vi "Folders_Required.vi"(1 "No dialogs":bool, 2 "Filenames":path[](array[path]), 3 "Add _pp?":bool, 4 "New Root":path) -> (0 "Array":path[](array[path]))   [LabVIEW 2012]
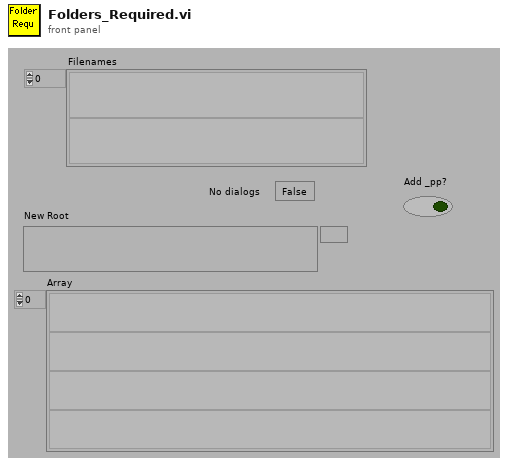
[diagram p1: front panel]
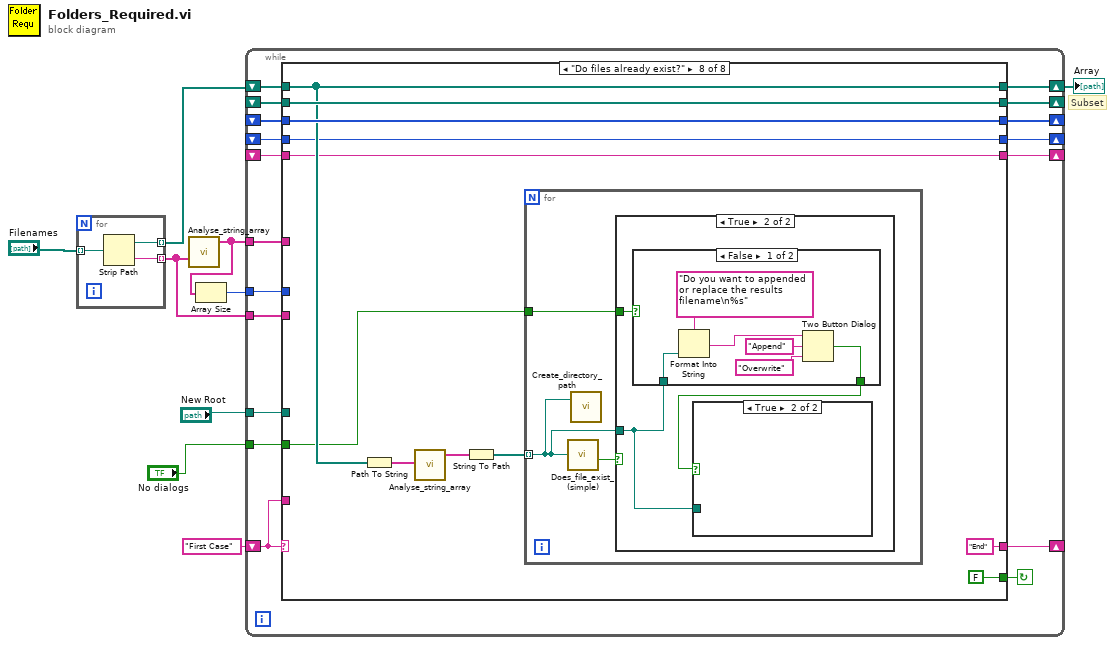
[diagram p0: block diagram]
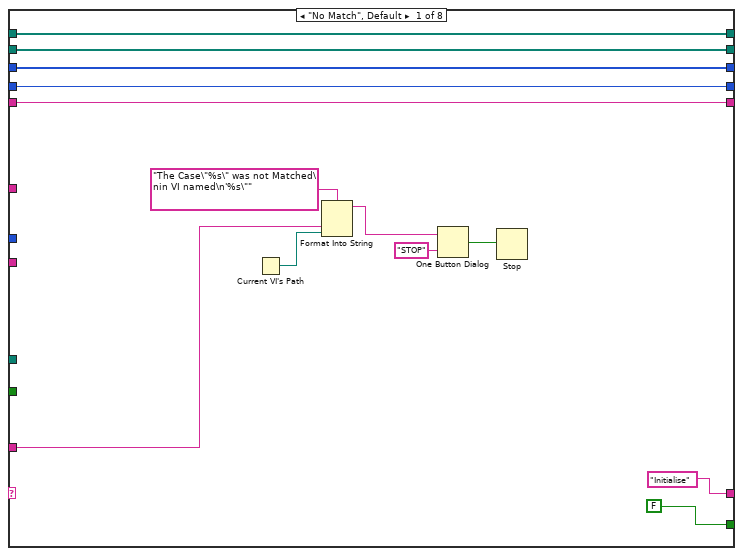
[diagram p2: hidden frame]
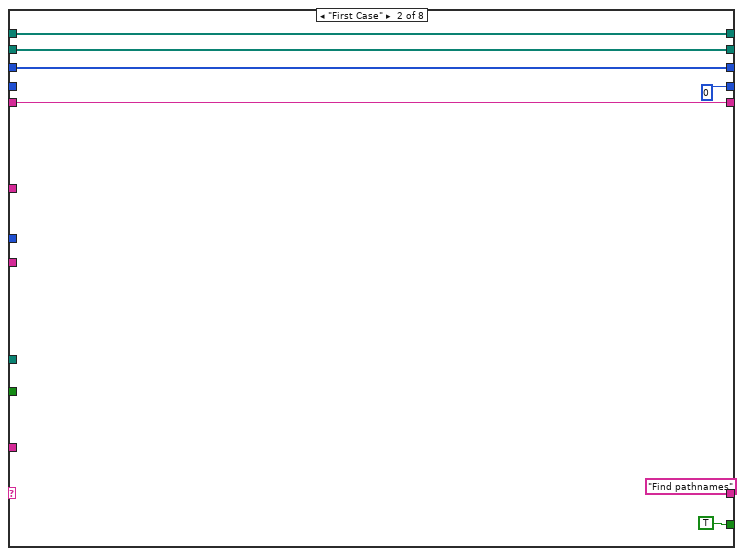
[diagram p3: hidden frame]
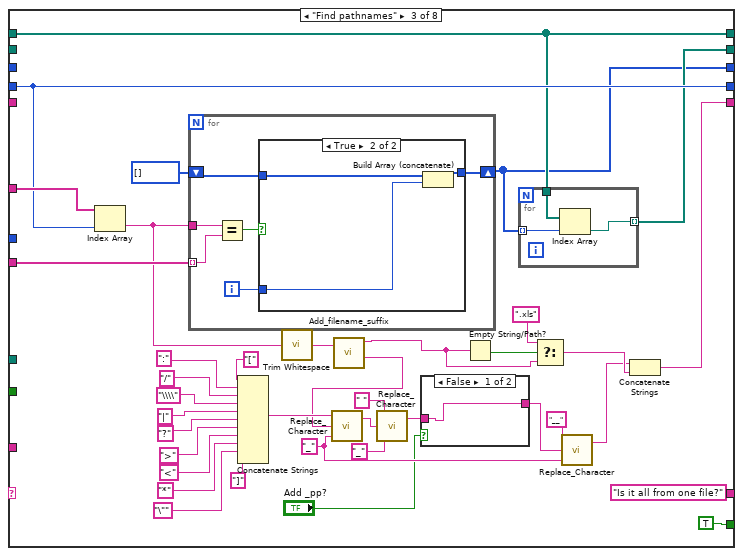
[diagram p4: hidden frame]
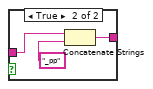
[diagram p5: hidden frame]
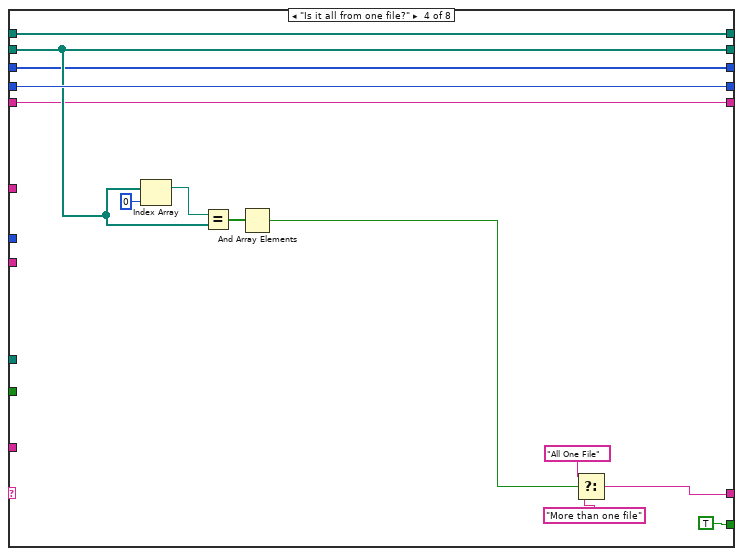
[diagram p7: hidden frame]
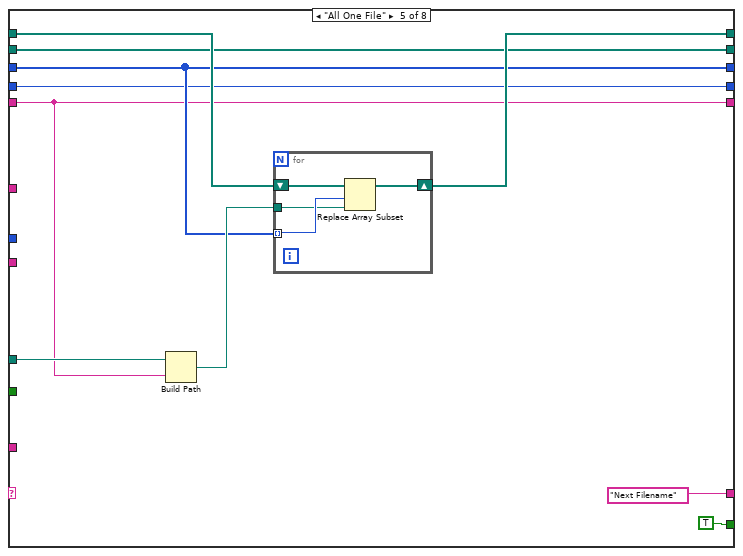
[diagram p8: hidden frame]
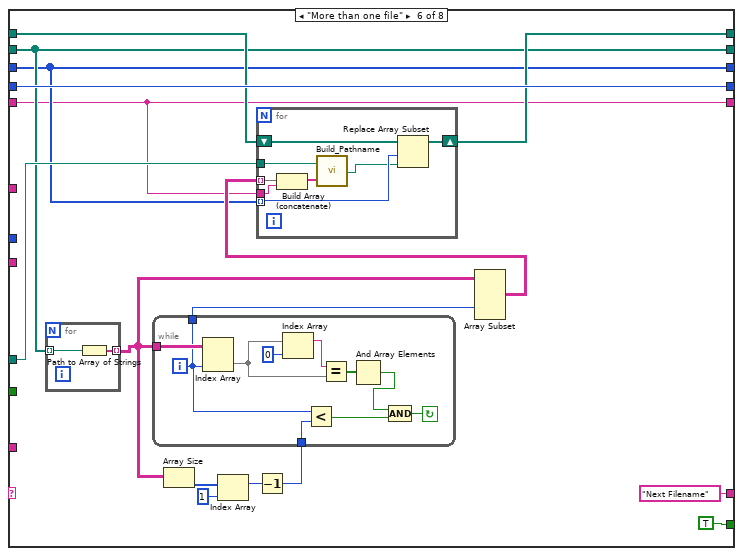
[diagram p9: hidden frame]
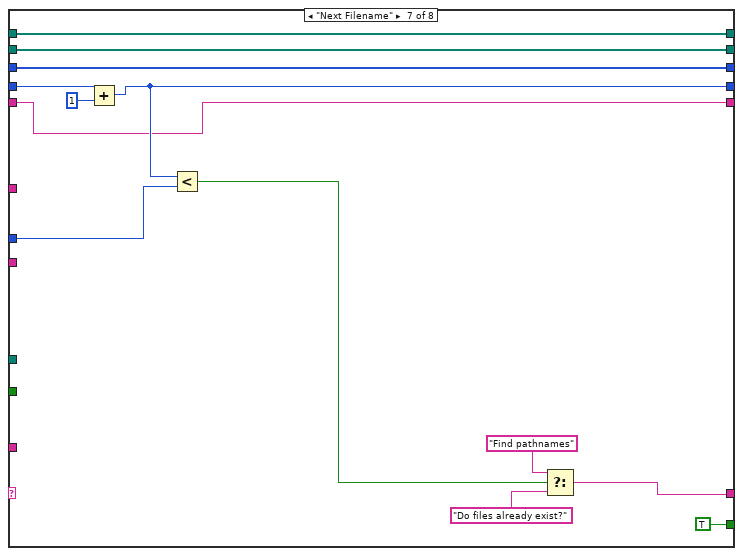
[diagram p10: hidden frame]
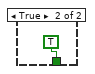
[diagram p12: hidden frame]
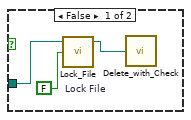
[diagram p13: hidden frame]
diagram:
  # "Subset"
  n1 = for {
    tunnel: "Filenames" -> [w12] mode=indexing
    tunnel: [w11] -> w8 mode=indexing
    tunnel: [w10] -> w2 mode=indexing
    n2 = Strip Path(path=w12) -> (stripped path=w10:path, name=w11:string)
  }
  n3 = call "Analyse_string_array.vi"("String array"=w8) -> ("Unique strings"=w6:string[])  [unwired: 2 out]
  n4 = Array Size(array=w6) -> (size(s)=w5:i32)
  n5 = while {
    shift-left: _ -> [w15]
    shift-right: [w14] -> _
    tunnel: w5 -> [w17]
    shift-left: w2 -> [w19]
    shift-right: [w20] -> w4
    tunnel: "New Root" -> [w21]
    tunnel: w8 -> [w22]
    tunnel: w6 -> [w23]
    shift-left: _ -> [w24]
    shift-right: [w26] -> _
    shift-left: _ -> [w25]
    shift-right: [w16] -> _
    shift-left: _ -> [w18]
    shift-right: [w27] -> _
    shift-left: "First Case" -> [w28]
    shift-right: [w29] -> _
    tunnel: "No dialogs" -> [w13]
    stop <- w30 continue-if-true
    n6 = case shown="\"Do files already exist?\"" w28 {
      tunnel: [FALSE TRUE TRUE TRUE TRUE TRUE TRUE FALSE] -> w30
      tunnel: ["Initialise" "Find pathnames" "Is it all from one file?" w113 "Next Filename" "Next Filename" w172 "End"] -> w29
      tunnel: w28 -> [w38 _ _ _ _ _ _ _]
      tunnel: [w34 w46 w81 w108 w123 w136 w181 w192] -> w27
      tunnel: [w33 0 w84 w117 w120 w147 w177 w186] -> w26
      tunnel: w25 -> [w32 w45 _ w107 w122 w135 w175 w191]
      tunnel: w24 -> [w33 _ w84 w117 w120 w147 w179 w186]
      tunnel: w23 -> [_ _ w86 _ _ _ _ _]
      tunnel: w22 -> [_ _ w85 _ _ _ _ _]
      tunnel: w21 -> [_ _ _ _ w127 w140 _ _]
      tunnel: [w35 w47 w82 w109 w124 w141 w180 w189] -> w20
      tunnel: w19 -> [w35 w47 w82 w109 w125 w142 w180 w189]
      tunnel: w18 -> [w34 w46 _ w108 w123 w136 w181 w192]
      tunnel: w17 -> [_ _ _ _ _ _ w176 _]
      tunnel: [w32 w45 w80 w107 w122 w135 w175 w191] -> w16
      tunnel: w15 -> [w31 w44 _ w106 w119 w133 w169 w184]
      tunnel: [w31 w44 w64 w106 w119 w133 w169 w184] -> w14
      tunnel: w13 -> [_ _ _ _ _ _ _ w182]
      frame "No Match", Default {
        n7 = Current VI's Path() -> (path=w37:path)
        n8 = Format Into String(format string="The Case\"%s\" was not Matched\nin VI named\n'%s\"" ("Format String"), w38, w37) -> (resulting string=w41:string)  [unwired: 2 in, 1 out]
        n9 = One Button Dialog(message=w41, button name ("OK")="STOP") -> (true=w39:bool)
        n10 = Stop(stop? (T)=w39) -> ()
      }
      frame "First Case" {
      }
      frame "Find pathnames" {
        w63 = "_" ("Replace with")
        n11 = Index Array(array=w86, index=w84) -> (element=w67:string)
        n12 = for {
          tunnel: w67 -> [w101]
          tunnel: w85 -> [w100] mode=indexing
          shift-right: [w97] -> w80
          shift-left: i32[] [] -> [w98]
          i -> [w96]
          n13 = Equal?(x=w101, y=w100) -> (x = y?=w99:bool)
          n14 = case shown="True" w99 {
            tunnel: w98 -> [w102 w105]
            tunnel: [w102 w104] -> w97
            tunnel: w96 -> [_ w103]
            frame False {
            }
            frame True {
              n15 = Build Array (concatenate)(w105, w103) -> (w104:i32[])
            }
          }
        }
        n16 = Concatenate Strings("[" ("Substring"), ":", "/", "\\\\", "|", "?", ">", "<", "*", "\"", "]" ("Substring")) -> (w68:string)
        n17 = call <vilib>:"Trim Whitespace.vi"("string"=w67) -> ("trimmed string"=w66:string)  [unwired: 1 in]
        n18 = call "Add_filename_suffix.vi"("Filename"=w66) -> ("Original Suffix"=w55:string, "Base name"=w65:string)  [unwired: 1 in, 2 out]
        n19 = call "Replace_Character.vi"("Replace with"=w63, "Input String"=w65, "Search For"=w68) -> ("Output string"=w59:string)  [unwired: 1 out]
        n20 = call "Replace_Character.vi"("Replace with"="_", "Input String"=w59, "Search For"=" ") -> ("Output string"=w60:string)  [unwired: 1 out]
        n21 = case shown="False" "Add _pp?" {
          tunnel: [w89 w91] -> w62
          tunnel: w60 -> [w89 w90]
          frame False {
          }
          frame True {
            n22 = Concatenate Strings(w90, "_pp" ("Substring")) -> (w91:string)
          }
        }
        n23 = Empty String/Path?(string/path=w55) -> (empty?=w56:bool)
        n24 = for {
          tunnel: w80 -> [w95] mode=indexing
          tunnel: w82 -> [w94]
          tunnel: [w93] -> w81 mode=indexing
          n25 = Index Array(array=w94, index=w95) -> (element=w93:path)
        }
        n26 = Select(t=".xls", s=w56, f=w55) -> (s? t:f=w54:string)
        n27 = call "Replace_Character.vi"("Replace with"=w63, "Input String"=w62, "Search For"="__") -> ("Output string"=w52:string)  [unwired: 1 out]
        n28 = Concatenate Strings(w52, w54) -> (w64:string)
      }
      frame "Is it all from one file?" {
        n29 = Index Array(array=w108, index=0 ("Index")) -> (element=w111:path)
        n30 = Equal?(x=w111, y=w108) -> (x = y?=w110:bool[])
        n31 = And Array Elements(Boolean array=w110) -> (logical AND=w116:bool)
        n32 = Select(t="All One File", s=w116, f="More than one file") -> (s? t:f=w113:string)
      }
      frame "All One File" {
        n33 = Build Path(base path=w127, name or relative path=w119) -> (appended path=w126:path)
        n34 = for {
          tunnel: w122 -> [w130] mode=indexing
          shift-right: [w131] -> w124
          shift-left: w125 -> [w132]
          tunnel: w126 -> [w129]
          n35 = Replace Array Subset(array=w132, new element=w129, index=w130) -> (w131:path[])
        }
      }
      frame "More than one file" {
        n36 = for {
          tunnel: w136 -> [w168] mode=indexing
          tunnel: [w167] -> w138 mode=indexing
          n37 = Path to Array of Strings(0:w168) -> (2:w167:string[])  [unwired: 1 out]
        }
        n38 = Array Size(array=w138) -> (size(s)=w145:i32[])
        n39 = Index Array(array=w145, index=1 ("Index")) -> (element=w144:i32)
        n40 = Decrement(x=w144) -> (x-1=w143:i32)
        n41 = while {
          tunnel: [w149] -> w139
          tunnel: w143 -> [w153]
          tunnel: w138 -> [w158]
          i -> [w149]
          stop <- w150 continue-if-true
          n42 = Index Array(array=w158, index (col)=w149) -> (element=w154:string[])  [unwired: 1 in]
          n43 = Index Array(array=w154, index=0 ("Index")) -> (element=w156:string)
          n44 = Less?(x=w149, y=w153) -> (x < y?=w152:bool)
          n45 = Equal?(x=w156, y=w154) -> (x = y?=w155:bool[])
          n46 = And Array Elements(Boolean array=w155) -> (logical AND=w151:bool)
          n47 = Compound Arithmetic op=AND(w151, w152) -> (w150:bool)
        }
        n48 = Array Subset(array=w138, index (col)=w139) -> (w137:string[][])  [unwired: 3 in]
        n49 = for {
          tunnel: w135 -> [w164] mode=indexing
          shift-right: [w165] -> w141
          shift-left: w142 -> [w166]
          tunnel: w140 -> [w163]
          tunnel: w137 -> [w161] mode=indexing
          tunnel: w133 -> [w159]
          n50 = Build Array (concatenate)(w161, w159) -> (w160:string[])
          n51 = call "Build_Pathname.vi"("PathElements"=w160, "PathnameIn"=w163) -> ("AppendedPath"=w162:path)
          n52 = Replace Array Subset(array=w166, new element=w162, index=w164) -> (w165:path[])
        }
      }
      frame "Next Filename" {
        n53 = Add(x=w179, y=1) -> (x+y=w177:i32)
        n54 = Less?(x=w177, y=w176) -> (x < y?=w174:bool)
        n55 = Select(t="Find pathnames", s=w174, f="Do files already exist?") -> (s? t:f=w172:string)
      }
      frame "Do files already exist?" {
        n56 = Path To String(path=w189) -> (string=w188:string[])
        n57 = call "Analyse_string_array.vi"("String array"=w188) -> ("Unique strings"=w183:string[])  [unwired: 2 out]
        n58 = String To Path(string=w183) -> (path=w187:path[])
        n59 = for {
          tunnel: w187 -> [w194] mode=indexing
          tunnel: w182 -> [w193]
          n60 = call "Does_file_exist_(simple).vi"("Pathname"=w194) -> ("exists?"=w195:bool)
          n61 = call "Create_directory_path.vi"("Path name"=w194) -> ()  [unwired: 1 in, 2 out]
          n62 = case shown="True" w195 {
            tunnel: w194 -> [_ w197]
            tunnel: w193 -> [_ w196]
            frame False {
            }
            frame True {
              n63 = case shown="False" w196 {
                tunnel: [w200 TRUE ("T button?")] -> w198
                tunnel: w197 -> [w199 _]
                frame False {
                  n64 = Format Into String(format string="Do you want to appended or replace the results filename\n%s" ("Format String"), w199) -> (resulting string=w203:string)  [unwired: 2 in, 1 out]
                  n65 = Two Button Dialog(message=w203, 1:"Overwrite" ("F button name (\"Cancel\")"), 2:"Append" ("T button name (\"OK\")")) -> (T button?=w200:bool)
                }
                frame True {
                }
              }
              n66 = case shown="True" w198 {
                tunnel: w197 -> [w208 _]
                frame False {
                  w207 = FALSE  # Lock File
                  n67 = call "Lock_File.vi"("Lock File"=w207, "path"=w208) -> ("dup path"=w206:path)  [unwired: 1 in, 2 out]
                  n68 = call "Delete_with_Check.vi"("FilePath"=w206) -> ()  [unwired: 1 out]
                }
                frame True {
                }
              }
            }
          }
        }
      }
    }
  }
  "Array" <- w4
